vi "Arm_Move_Command.vi"(11 "Argument":dbl) -> ()   [LabVIEW 2014]
uses:
  TORC Code/GlobalVariable.vi
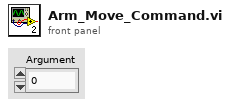
[diagram p1: front panel]
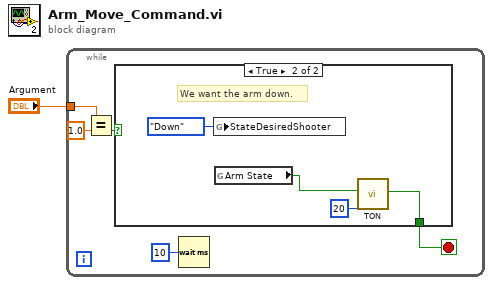
[diagram p0: block diagram]
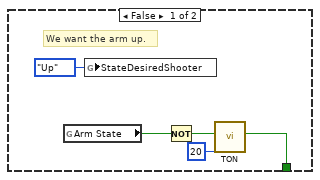
[diagram p2: hidden frame]
diagram:
  n1 = while {
    tunnel: "Argument" -> [w5]
    stop <- w2 stop-if-true
    n2 = Equal?(x=w5, y=1.0) -> (x = y?=w6:bool)
    n3 = case shown="True" w6 {
      tunnel: [w9 w14] -> w2
      frame False {
        # "We want the arm up."
        n4 = global read "GlobalVariable.vi" "Arm State"() -> (w11:bool)
        n5 = global write "GlobalVariable.vi" "StateDesiredShooter"(enum16{"None", "Down", "Up"}."Up" ("StateDesiredShooter")) -> ()
        n6 = Not(x=w11) -> (.not. x?=w8:bool)
        n7 = call "TON.vi"("Delay (ms)"=u32 20 ("Delay ms"), "Input"=w8) -> ("Output"=w9:bool)  [unwired: 9 in]
      }
      frame True {
        # "We want the arm down."
        n8 = global write "GlobalVariable.vi" "StateDesiredShooter"(enum16{"None", "Down", "Up"}."Down" ("StateDesiredShooter")) -> ()
        n9 = global read "GlobalVariable.vi" "Arm State"() -> (w13:bool)
        n10 = call "TON.vi"("Delay (ms)"=u32 20 ("Delay ms"), "Input"=w13) -> ("Output"=w14:bool)  [unwired: 9 in]
      }
    }
    n11 = Wait (ms)(milliseconds to wait=u32 10) -> ()  [unwired: 1 out]
  }
